vi "DRWM_DSF.vi"(5 "棒限值":dbl[](array[numeric]), 6 "DSF因子":cluster{"x":dbl, "y":dbl}[][](array[cluster]), 7 "DRWM开":bool, 8 "动态棒位":dbl, 10 "上下段通量选择":u16[](array[numeric]), 11 "反应性in":dbl[](array[numeric])) -> (3 "反应性out":dbl[](array[numeric]))   [LabVIEW 2020]
uses:
  <vilib>/Analysis/baseanly.llb/Mean (DBL).vi
  <vilib>/Analysis/NI_AALBase.lvlib
panel:
  out "下段":dbl caption="下段降棒前正反应性" format="%0.2f"
  out "上段":dbl caption="上段降棒前正反应性" format="%0.2f"
  out "下段测量总价值":dbl format="%0.2f"
  out "上段测量总价值":dbl format="%0.2f"
  out "反应性积累":dbl[][](array[numeric])
  out "棒位积累":dbl[](array[numeric])
  out "价值曲线":cluster{dbl[], dbl[]}[](graph) caption="（X和Y数组）多曲线"
  in  "棒位到底":bool
  in  "落棒前正反应性":dbl[][](array[numeric])
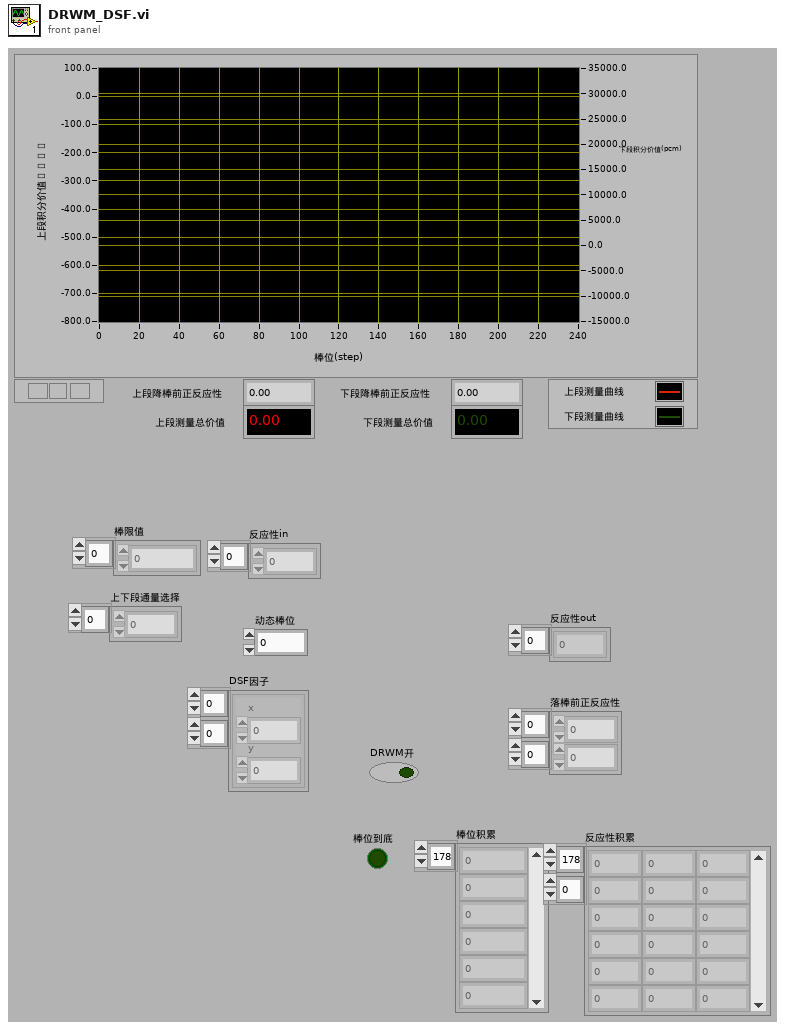
[diagram p1: front panel]
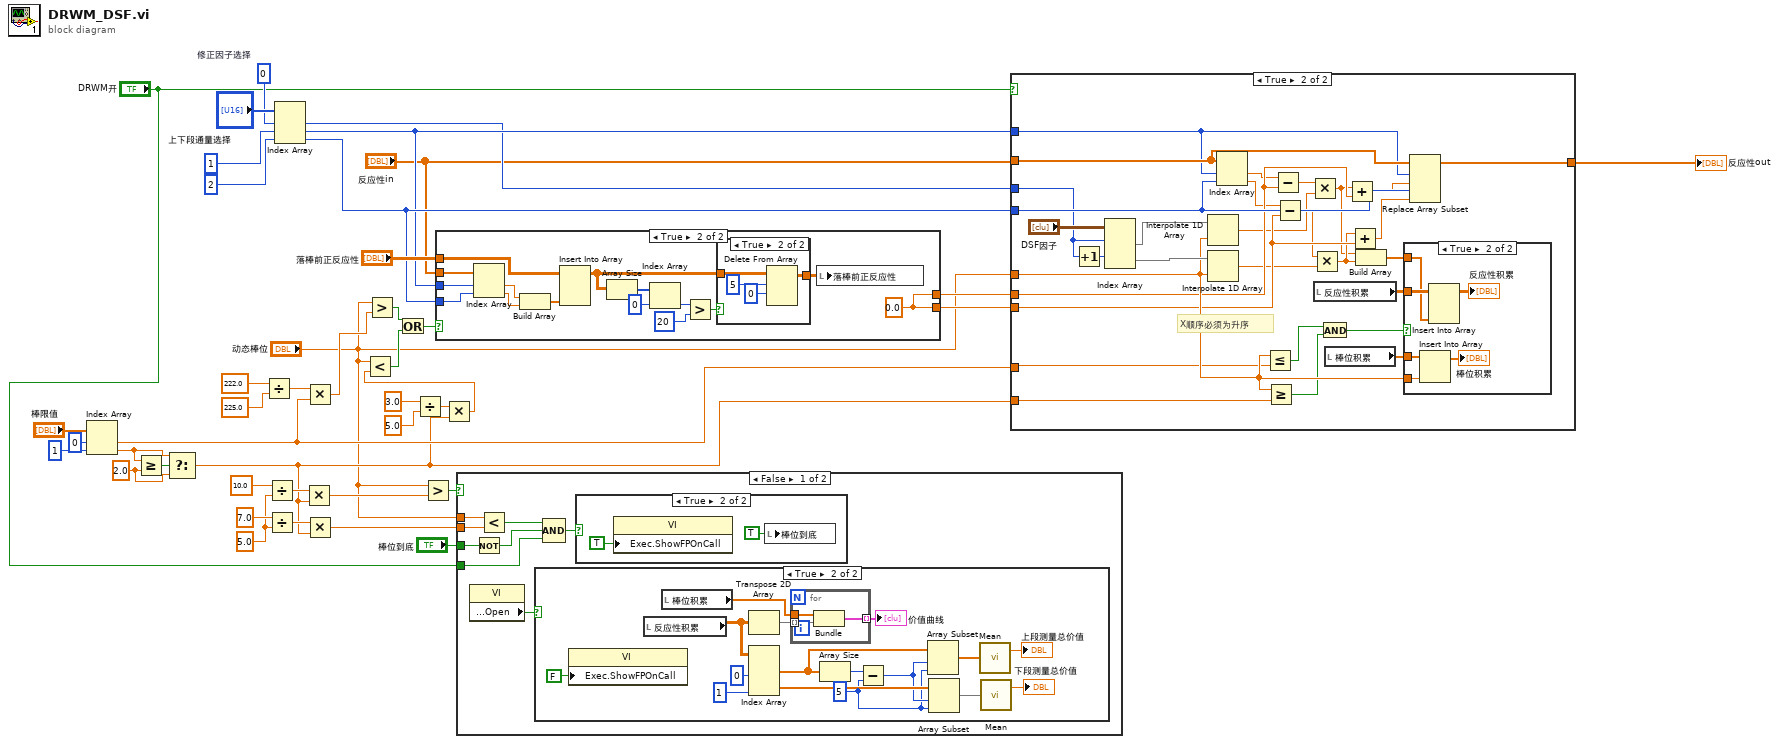
[diagram p0: block diagram]
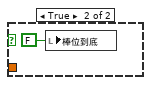
[diagram p4: hidden frame]
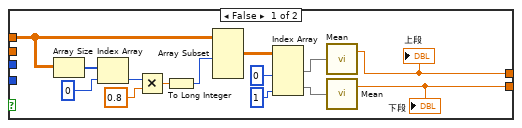
[diagram p5: hidden frame]
diagram:
  w11 = 2.0 ("y")
  w15 = 0  # 修正因子选择
  w10 = 5.0 ("y")
  n1 = Index Array(array="棒限值", index #1=0 ("索引"), index #2=1 ("索引")) -> (element #1=w31:dbl, element #2=w12:dbl)
  n2 = Greater Or Equal?(x=w12, y=w11) -> (x >= y?=w14:bool)
  n3 = Select(t=w12, s=w14, f=w11) -> (s? t:f=w13:dbl)
  n4 = Divide(x=222.0, y=225.0) -> (x/y=w30:dbl)
  n5 = Divide(x=10.0, y=w10) -> (x/y=w22:dbl)
  n6 = Divide(x=7.0, y=w10) -> (x/y=w20:dbl)
  n7 = Index Array(array="上下段通量选择", index #1=w15, index #2=1 ("索引"), index #3=2 ("索引")) -> (element #1=w6:u16, element #2=w7:u16, element #3=w8:u16)
  n8 = Multiply(x=w22, y=w13) -> (x*y=w18:dbl)
  n9 = Multiply(x=w30, y=w31) -> (x*y=w27:dbl)
  n10 = Multiply(x=w20, y=w13) -> (x*y=w17:dbl)
  n11 = Greater?(x="动态棒位", y=w27) -> (0:w39:bool)
  n12 = Divide(x=3.0, y=5.0) -> (x/y=w26:dbl)
  n13 = Greater?(x="动态棒位", y=w18) -> (0:w36:bool)
  n14 = Multiply(x=w26, y=w13) -> (x*y=w23:dbl)
  n15 = Less?(x="动态棒位", y=w23) -> (x < y?=w38:bool)
  n16 = Or(x=w39, y=w38) -> (x .or. y?=w37:bool)
  n17 = case shown="True" w37 {
    tunnel: "反应性in" -> [_ w71]
    tunnel: w7 -> [_ w70]
    tunnel: w8 -> [_ w69]
    tunnel: "落棒前正反应性" -> [w56 w58]
    tunnel: [w44 w57] -> w41
    tunnel: [w43 w57] -> w40
    frame False {
      n18 = Array Size(array=w56) -> (size(s)=w55:i32[])
      n19 = Index Array(array=w55, index=0 ("索引")) -> (element=w53:i32)
      n20 = Multiply(x=w53, y=0.8 ("元素")) -> (x*y=w51:dbl)
      n21 = To Long Integer(number=w51) -> (32bit integer=w50:i32)
      n22 = Array Subset(array=w56, length (row)=w50) -> (w49:dbl[][])  [unwired: 3 in]
      n23 = Index Array(array=w49, index (col) #1=0 ("禁用的索引 (列)"), index (col) #2=1 ("索引 (列)")) -> (element #1=w46:dbl[], element #2=w45:dbl[])  [unwired: 2 in]
      n24 = call-poly <vilib>:"Mean.vi"("X"=w46) -> ("mean"=w44:dbl)  [unwired: 1 out]
      "上段" <- w44
      n25 = call-poly <vilib>:"Mean.vi"("X"=w45) -> ("mean"=w43:dbl)  [unwired: 1 out]
      "下段" <- w43
    }
    frame True {
      w57 = 0.0 ("mean")
      n26 = Index Array(array=w71, index #1=w70, index #2=w69) -> (element #1=w68:dbl, element #2=w67:dbl)
      n27 = Build Array(w68, w67) -> (w66:dbl[])
      n28 = Insert Into Array(array=w58, new element=w66) -> (w65:dbl[][])  [unwired: 2 in]
      n29 = Array Size(array=w65) -> (size(s)=w63:i32[])
      n30 = Index Array(array=w63, index=0 ("索引")) -> (element=w61:i32)
      n31 = Greater?(x=w61, y=20) -> (0:w59:bool)
      n32 = case shown="True" w59 {
        tunnel: w65 -> [w72 w76]
        tunnel: [w72 w75] -> w64
        frame False {
        }
        frame True {
          n33 = Delete From Array(array=w76, length=5 ("长度"), index (row)=0 ("索引 (行)")) -> (array with subset deleted=w75:dbl[][])  [unwired: 1 in, 1 out]
        }
      }
      n34 = local write "落棒前正反应性"(w64) -> ()
    }
  }
  n35 = case shown="False" w36 {
    tunnel: "动态棒位" -> [w84 _]
    tunnel: "棒位到底" -> [w83 _]
    tunnel: w17 -> [w81 _]
    tunnel: "DRWM开" -> [w77 _]
    frame False {
      n36 = property class="VI"() -> ("Front Panel.Open"=w82:bool)  [unwired: 2 in, 2 out]
      n37 = Not(x=w83) -> (.not. x?=w79:bool)
      n38 = Less?(x=w84, y=w81) -> (x < y?=w80:bool)
      n39 = case shown="True" w82 {
        frame False {
        }
        frame True {
          w85 = 5 ("y")
          n40 = property class="VI"("Exec.ShowFPOnCall"=FALSE ("执行:调用时显示前面板")) -> ()  [unwired: 2 in, 2 out]
          n41 = local read "反应性积累"() -> (w96:dbl[][])
          n42 = local read "棒位积累"() -> (w98:dbl[])
          n43 = Transpose 2D Array(2D array=w96) -> (transposed array=w97:dbl[][])
          n44 = Index Array(array=w96, index (col) #1=0 ("禁用的索引 (列)"), index (col) #2=1 ("索引 (列)")) -> (element #1=w88:dbl[], element #2=w89:dbl[])  [unwired: 2 in]
          n45 = for {
            tunnel: w98 -> [w101]
            tunnel: w97 -> [w102] mode=indexing
            tunnel: [w103] -> w99 mode=indexing
            n46 = Bundle "Bundle"("棒位积累"=w101, w102) -> (w103:cluster{"棒位积累":dbl[], dbl[]})  [unwired: 1 in]
          }
          "价值曲线" <- w99
          n47 = Array Size(array=w88) -> (size(s)=w87:i32)
          n48 = Subtract(x=w87, y=w85) -> (x-y=w86:i32)
          n49 = Array Subset(array=w88, index=w86, length=w85) -> (w93:dbl[])
          n50 = Array Subset(array=w89, index=w86, length=w85) -> (w92:dbl[])
          n51 = call-poly <vilib>:"Mean.vi"("X"=w93) -> ("mean"=→"上段测量总价值":dbl)  [unwired: 1 out]
          n52 = call-poly <vilib>:"Mean.vi"("X"=w92) -> ("mean"=→"下段测量总价值":dbl)  [unwired: 1 out]
        }
      }
      n53 = Compound Arithmetic op=AND(w80, w79, w77) -> (w78:bool)
      n54 = case shown="True" w78 {
        frame False {
        }
        frame True {
          n55 = property class="VI"("Exec.ShowFPOnCall"=TRUE ("执行:调用时显示前面板")) -> ()  [unwired: 2 in, 2 out]
          n56 = local write "棒位到底"(TRUE ("棒位到底")) -> ()
        }
      }
    }
    frame True {
      n57 = local write "棒位到底"(FALSE ("棒位到底")) -> ()
    }
  }
  n58 = case shown="True" "DRWM开" {
    tunnel: [w107 w137] -> w1
    tunnel: "反应性in" -> [w107 w133]
    tunnel: "动态棒位" -> [_ w132]
    tunnel: w8 -> [_ w131]
    tunnel: w7 -> [_ w130]
    tunnel: w41 -> [_ w129]
    tunnel: w40 -> [_ w128]
    tunnel: w31 -> [_ w127]
    tunnel: w13 -> [_ w126]
    tunnel: w6 -> [_ w124]
    frame False {
    }
    frame True {
      # "X顺序必须为升序"
      n59 = Increment(x=w124) -> (x+1=w125:u16)
      n60 = Index Array(array="DSF因子", index (row) #1=w124, index (row) #2=w125) -> (element #1=w135:cluster{"x":dbl, "y":dbl}[], element #2=w134:cluster{"x":dbl, "y":dbl}[])  [unwired: 2 in]
      n61 = Interpolate 1D Array(1:w132, 2:w135) -> (0:w123:dbl)
      n62 = Interpolate 1D Array(1:w132, 2:w134) -> (0:w122:dbl)
      n63 = Index Array(array=w133, index #1=w130, index #2=w131) -> (element #1=w121:dbl, element #2=w120:dbl)
      n64 = Less Or Equal?(x=w132, y=w127) -> (x <= y?=w110:bool)
      n65 = Greater Or Equal?(x=w132, y=w126) -> (x >= y?=w111:bool)
      n66 = Subtract(x=w121, y=w129) -> (x-y=w118:dbl)
      n67 = Subtract(x=w120, y=w128) -> (x-y=w119:dbl)
      n68 = Multiply(x=w118, y=w123) -> (x*y=w108:dbl)
      n69 = Multiply(x=w119, y=w122) -> (x*y=w109:dbl)
      n70 = local read "反应性积累"() -> (w114:dbl[][])
      n71 = And(x=w110, y=w111) -> (x .and. y?=w112:bool)
      n72 = local read "棒位积累"() -> (w115:dbl[])
      n73 = Add(x=w108, y=w129) -> (x+y=w117:dbl)
      n74 = Add(x=w109, y=w128) -> (x+y=w116:dbl)
      n75 = Build Array(w108, w109) -> (w113:dbl[])
      n76 = case shown="True" w112 {
        tunnel: w115 -> [_ w143]
        tunnel: w132 -> [_ w141]
        tunnel: w114 -> [_ w139]
        tunnel: w113 -> [_ w138]
        frame False {
        }
        frame True {
          n77 = Insert Into Array(array=w143, new element=w141) -> (→"棒位积累":dbl[])  [unwired: 1 in]
          n78 = Insert Into Array(array=w139, new element=w138) -> (→"反应性积累":dbl[][])  [unwired: 2 in]
        }
      }
      n79 = Replace Array Subset(array=w133, new element #1=w117, index #1=w130, new element #2=w116, index #2=w131) -> (w137:dbl[])
    }
  }
  "反应性out" <- w1
